vi "workbook close.vi"(8 "error in (no error)":errorcluster, 11 "workbook":u32) -> (0 "error out":errorcluster, 3 "function return":u32(ring))   [LabVIEW 2015, in "xlsxwriter.lvlib"]
doc: "lxw_error workbook_close(lxw_workbook workbook);"
uses:
  xlsxwriter.lvlib
  xlsxwriter.dll
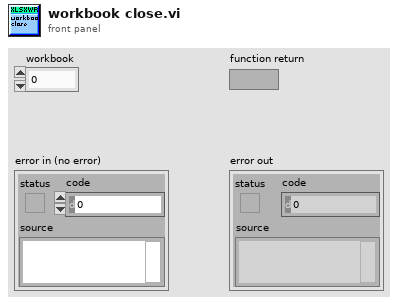
[diagram p1: front panel]
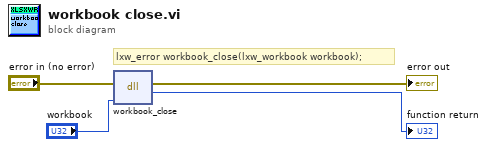
[diagram p0: block diagram]
diagram:
  # "lxw_error workbook_close(lxw_workbook workbook);"
  n1 = dll-call lib="C:/Users/WDAGUtilityAccount/Desktop/lv_vis_added_cell/xlsxwriter.*" fn="workbook_close"(error in="error in (no error)", "workbook"="workbook") -> (error out=→"error out":errorcluster, →"function return":u32)  [unwired: 3 in, 1 out]
